vi "getViInformation.vi"() -> ()   [LabVIEW 2017, in "vi_tools.lvlib"]
doc: "Retrieves the information from the active VI"
uses:
  vi_tools.lvlib
  connectorPanePatterns.ctl
  shared/shared.lvlib
panel:
  in  "Tab Control":enum32{"General", "Documentation", "Execution"}(tab)
  out "ConPane Pattern":T1=3
  out "Icon":picture
  out "VI Revision":u32
  out "History":string
  out "Source Version":string
  out "SeparateCompiledCode":bool caption="Compiled code separated from source file"
  out "Path":path
  out "Name":string
  in  "Bookmarks":i32(listbox)
  out "Help path/URL":string
  out "Help Tag":string
  out "Description":string
  out "Suspend when called":bool
  out "Automatic error handling":bool
  out "Run when opened":bool
  out "Reentrancy Type":T2(ring)
  out "Priority":T3(ring)
  out "Preferred Exec System":T4(ring)
  out "Is Reentrant":bool
  out "Allow Debugging":bool
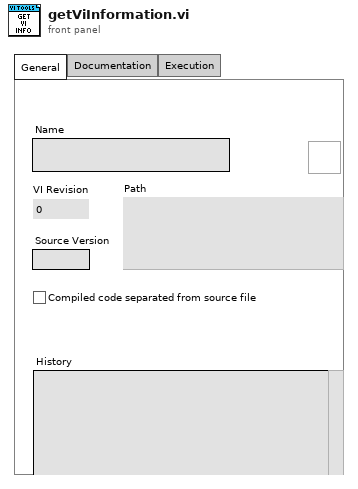
[diagram p1: front panel]
types:
  T1 = typedef "vi_tools.lvlib/connectorPanePatterns.ctl" = i32
  T2 = enum16{"Share clones between instances", "Preallocate clone for each instance"}
  T3 = enum32{"invalid priority", "background priority", "normal priority", "above normal priority", "high priority", "time critical priority", "subroutine"}
  T4 = enum32{"invalid execution system", "user interface", "standard", "instrument i/o", "data acquisition", "other 1", "other 2", "same as caller"}
  T5 = enum32{"Invalid", "Standard", "Closed", "Hidden", "Minimized", "Maximized"}
  T6 = cluster{"VI Name":string, "VI Path":path, "VI Revision":u32, "VI History":string, "CompileCodeSeparated":bool, "VI Version":cluster{"VI Version":string, "VI Vers":u32, "VI Editor Version":string, "VI Editor Vers":u32}, "ConPane Pattern":T1, "Icon Image":picture}
  T7 = cluster{"VI Description":string, "VI Help.Tag":string, "VI Help.Doc":string}
  T8 = cluster{"AllowDebugging":bool, "IsReentrant":bool, "ReentrancyType":enum16{"Share clones between instances", "Preallocate clone for each instance"}, "PrefSys":enum32{"invalid execution system", "user interface", "standard", "instrument i/o", "data acquisition", "other 1", "other 2", "same as caller"}, "riority":enum32{"invalid priority", "background priority", "normal priority", "above normal priority", "high priority", "time critical priority", "subroutine"}, "RunOnOpen":bool, "Def Err Handling":bool, "SuspOnCall":bool}
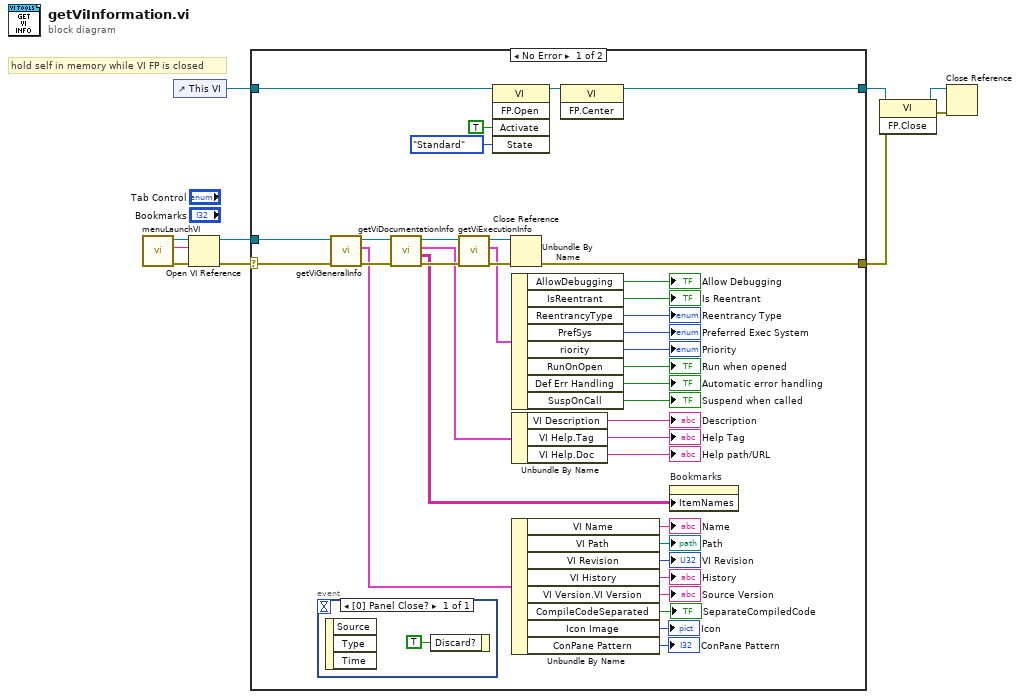
[diagram p0: block diagram]
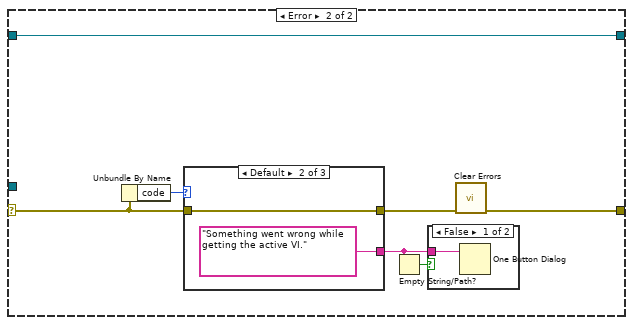
[diagram p2: hidden frame]
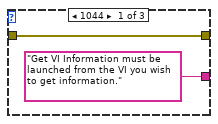
[diagram p4: hidden frame]
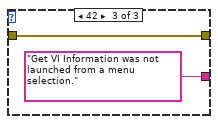
[diagram p5: hidden frame]
diagram:
  # "hold self in memory while VI FP is closed"
  n1 = call "menuLaunchVI.vi"() -> ("error out"=w8:errorcluster, "Menu Launch:VI"=w9:string, "Menu Launch:App"=w2:refnum<vi>)  [unwired: 9 in]
  n2 = control-ref of="This VI"() -> (w1:refnum<vi>)
  n3 = Open VI Reference(application reference (local)=w2, vi path=w9, error in (no error)=w8) -> (vi reference=w10:refnum<vi>, error out=w7:errorcluster)  [unwired: 3 in]
  n4 = case shown="No Error" w7 {
    selector: w7 -> [w40 w54]
    tunnel: [w47 w50] -> w6
    tunnel: w10 -> [w39 _]
    tunnel: w1 -> [w15 w49]
    tunnel: [w13 w49] -> w3
    frame No Error {
      n5 = event shown="[0] Panel Close?" {
        selector: _ -> [_]
        dyn-events: _ -> [_]
        timeout: _ -> [_]
        event Panel Close? {
          n6 = event-data() -> ()  [unwired: 1 in, 3 out]
          n7 = event-data("Discard?"=TRUE) -> ()  [unwired: 1 in, 1 out]
        }
      }
      n8 = call "getViGeneralInfo.vi"("error in (no error)"=w40, "VI in"=w39) -> ("error out"=w45:errorcluster, "VI General Info"=w16:T6, "VI out"=w46:refnum<vi>)  [unwired: 7 in]
      n9 = call "getViDocumentationInfo.vi"("error in (no error)"=w45, "VI in"=w46) -> ("error out"=w43:errorcluster, "Bookmarks"=w19:string[][], "VI Documentation Info"=w17:T7, "VI out"=w44:refnum<vi>)  [unwired: 6 in]
      n10 = call "getViExecutionInfo.vi"("error in (no error)"=w43, "VI in"=w44) -> ("error out"=w42:errorcluster, "VI Execution Info"=w18:T8, "VI out"=w41:refnum<vi>)  [unwired: 7 in]
      n11 = invoke class="VI" method="FP.Open"(reference=w15, "Activate"=TRUE ("Activate?"), "State"=T5."Standard") -> (reference out=w14:refnum<vi>)  [unwired: 2 in, 4 out]
      n12 = Close Reference(reference=w41, error in (no error)=w42) -> (error out=w47:errorcluster)
      n13 = Unbundle By Name(w18) -> ("AllowDebugging"=→"Allow Debugging":bool, "IsReentrant"=→"Is Reentrant":bool, "ReentrancyType"=→"Reentrancy Type":T2, "PrefSys"=→"Preferred Exec System":T4, "riority"=→"Priority":T3, "RunOnOpen"=→"Run when opened":bool, "Def Err Handling"=→"Automatic error handling":bool, "SuspOnCall"=→"Suspend when called":bool)
      n14 = Unbundle By Name(w17) -> ("VI Description"=→"Description":string, "VI Help.Tag"=→"Help Tag":string, "VI Help.Doc"=→"Help path/URL":string)
      n15 = Unbundle By Name(w16) -> ("VI Name"=→"Name":string, "VI Path"=→"Path":path, "VI Revision"=→"VI Revision":u32, "VI History"=→"History":string, "VI Version.VI Version"=→"Source Version":string, "CompileCodeSeparated"=→"SeparateCompiledCode":bool, "Icon Image"=→"Icon":picture, "ConPane Pattern"=→"ConPane Pattern":T1)
      n16 = invoke class="VI" method="FP.Center"(reference=w14) -> (reference out=w13:refnum<vi>)  [unwired: 2 in, 2 out]
      n17 = property on="Bookmarks" class="MCListbox (strict)"("ItemNames"=w19) -> ()  [unwired: 2 in, 2 out]
    }
    frame Error {
      n18 = Unbundle By Name(w54) -> ("code"=w55:i32)
      n19 = case shown="Default" w55 {
        tunnel: w54 -> [w58 w60 w62]
        tunnel: [w58 w60 w62] -> w51
        tunnel: ["Get VI Information must be launched from the VI you wish to get information." ("message") "Something went wrong while getting the active VI." ("message") "Get VI Information was not launched from a menu selection." ("message")] -> w53
        frame 1044 {
        }
        frame Default {
        }
        frame 42 {
        }
      }
      n20 = Empty String/Path?(string/path=w53) -> (empty?=w52:bool)
      n21 = case shown="False" w52 {
        tunnel: w53 -> [w56 _]
        frame False {
          n22 = One Button Dialog(message=w56) -> ()  [unwired: 1 in, 1 out]
        }
        frame True {
        }
      }
      n23 = call <vilib>:"Clear Errors.vi"("error in (no error)"=w51) -> ("error out"=w50:errorcluster)  [unwired: 5 in, 1 out]
    }
  }
  n24 = invoke class="VI" method="FP.Close"(reference=w3, error in=w6) -> (reference out=w4:refnum<vi>, error out=w5:errorcluster)  [unwired: 1 in, 1 out]
  n25 = Close Reference(reference=w4, error in (no error)=w5) -> ()  [unwired: 1 out]
